vi "read e-series ini file.vi"(8 "error in (no error)":errorcluster, 11 "ini filename":string) -> (0 "error out":errorcluster, 3 "File Names":string[](array[string]))   [LabVIEW 2018]
uses:
  <vilib>/Utility/config.llb/Read Key (String).vi
  <vilib>/Utility/config.llb/NI_LVConfig.lvlib
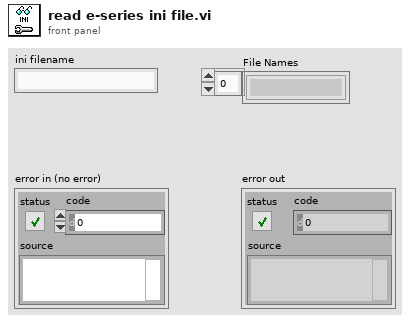
[diagram p1: front panel]
types:
  T1 = typedef "NI_LVConfig.lvlib/Config Data RefNum.ctl" = refnum<k1>
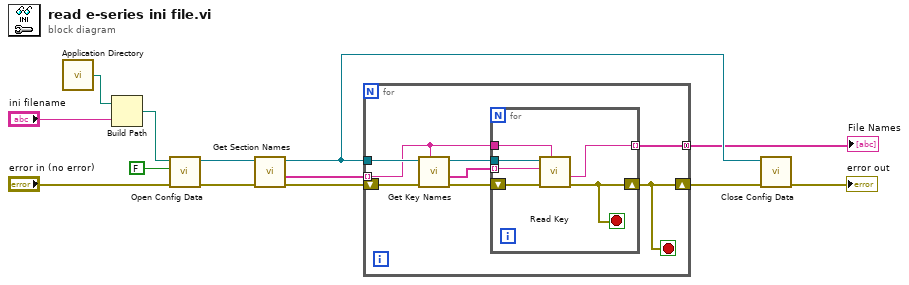
[diagram p0: block diagram]
diagram:
  n1 = call <vilib>:"Application Directory.vi"() -> ("Application Directory"=w12:path)
  n2 = Build Path(base path=w12, name or relative path="ini filename") -> (appended path=w10:path)
  n3 = call <vilib>:"Open Config Data.vi"("error in (no error)"="error in (no error)", "create file if necessary (T)"=FALSE, "configuration file path"=w10) -> ("error out"=w9:errorcluster, "refnum"=w7:T1)  [unwired: 6 in, 1 out]
  n4 = call <vilib>:"Get Section Names.vi"("error in (no error)"=w9, "refnum"=w7) -> ("error out"=w8:errorcluster, "section names"=w3:string[], "refnum out"=w4:T1)  [unwired: 7 in]
  n5 = for {
    shift-right: [w14] -> w2
    shift-left: w8 -> [w21]
    tunnel: w3 -> [w18] mode=indexing
    tunnel: w4 -> [w20]
    tunnel: [w16] -> w1 mode=concatenating
    stop <- w14 stop-if-true
    n6 = call <vilib>:"Get Key Names.vi"("section"=w18, "error in (no error)"=w21, "refnum"=w20) -> ("error out"=w19:errorcluster, "key names"=w17:string[], "refnum out"=w15:T1)  [unwired: 5 in, 1 out]
    n7 = for {
      shift-right: [w22] -> w14
      shift-left: w19 -> [w27]
      tunnel: w18 -> [w26]
      tunnel: w17 -> [w25] mode=indexing
      tunnel: [w24] -> w16 mode=indexing
      tunnel: w15 -> [w23]
      stop <- w22 stop-if-true
      n8 = call-poly <vilib>:"Read Key.vi"("section"=w26, "error in (no error)"=w27, "key"=w25, "refnum"=w23) -> ("error out"=w22:errorcluster, "value"=w24:string)  [unwired: 4 in, 2 out]
    }
  }
  "File Names" <- w1
  n9 = call <vilib>:"Close Config Data.vi"("error in (no error)"=w2, "refnum"=w4) -> ("error out"=→"error out":errorcluster)  [unwired: 8 in, 1 out]
